vi "NIIE_SET_ToolGraphic.vi"(8 "Error":errorcluster, 9 "Temp Coord":T5, 10 "Temp Icon":picture, 11 "Data":T1={"Class"={"Ants"=refnum, "Layer"=refnum, "Templates"=refnum, "Icon"=refnum, "Glyph"=refnum, "Settings"=refnum, "Tools"=refnum}, "Ref"={"Add Layer"=refnum, "Remove Layer"=refnum, "Line Text"=[], "Body Text Spec"=refnum, "DNL_Font"=refnum, "glyph path str"=refnum, "templates path str"=refnum, "Arrow Up"=refnum, "Arrow Down"=refnum, "IE VI Ref"=refnum, "Glyphs tree"=refnum, "Templates tree"=refnum, "Layer Icon Text"=refnum, "Layer Template"=refnum, "Clipboard"=refnum, "BW icon in"=refnum, "Color icon in"=refnum, "Layer Clust"=refnum, "Body Text"=refnum, "DNL_Framework Templates"=refnum, "Search Templates"=refnum, "TextMarker"=refnum, "Tab Control"=refnum, "Search Glyphs"=refnum, "Line Color"=refnum, "DNL_Glyphs []"=refnum, "Fill Color"=refnum, "Tools"=refnum, "Glyphs tree"=refnum, "Icon"=refnum, "Preview"=refnum, "Ants"=refnum, "Terminals"=refnum, "menu reference"=refnum, "LayerNames"=[], "GlyphLoadAnimation"=refnum, "TemplateLoadAnimation"=refnum, "refreshGlyphs"=refnum, "refreshTemplates"=refnum}, "Support"={"AntsRect"={"left"=0, "top"=0, "right"=0, "bottom"=0}, "Mouse Move Coords"={"Horizontal"=0, "Vertical"=0}, "Mouse Down Coords"={"Horizontal"=0, "Vertical"=0}, "Temp Coord"={"Horizontal"=0, "Vertical"=0}, "Action"=enum."Default", "Edge Color"=4914962, "Fill Color"=16860, "Mouse Down?"=FALSE, "Draft Mode?"=FALSE, "Temp Icon"=bytes[3102], "CTRL Pressed"=FALSE, "Move Selection?"=FALSE, "AntsRect Orig"={"left"=0, "top"=0, "right"=0, "bottom"=0}, "Text"="", "TM Set?"=FALSE, "Mouse inside icon?"=FALSE, "Tool (old value)"=0, "Pencil Move Color"=0, "Swap Colors?"=FALSE, "Shift pressed?"=FALSE}}) -> (0 "Error Out":errorcluster, 1 "All Layers Out":refnum<class "Layer.lvclass">[](array[class]), 3 "Data Out":T1={"Class"={"Ants"=refnum, "Layer"=refnum, "Templates"=refnum, "Icon"=refnum, "Glyph"=refnum, "Settings"=refnum, "Tools"=refnum}, "Ref"={"Add Layer"=refnum, "Remove Layer"=refnum, "Line Text"=[], "Body Text Spec"=refnum, "DNL_Font"=refnum, "glyph path str"=refnum, "templates path str"=refnum, "Arrow Up"=refnum, "Arrow Down"=refnum, "IE VI Ref"=refnum, "Glyphs tree"=refnum, "Templates tree"=refnum, "Layer Icon Text"=refnum, "Layer Template"=refnum, "Clipboard"=refnum, "BW icon in"=refnum, "Color icon in"=refnum, "Layer Clust"=refnum, "Body Text"=refnum, "DNL_Framework Templates"=refnum, "Search Templates"=refnum, "TextMarker"=refnum, "Tab Control"=refnum, "Search Glyphs"=refnum, "Line Color"=refnum, "DNL_Glyphs []"=refnum, "Fill Color"=refnum, "Tools"=refnum, "Glyphs tree"=refnum, "Icon"=refnum, "Preview"=refnum, "Ants"=refnum, "Terminals"=refnum, "menu reference"=refnum, "LayerNames"=[], "GlyphLoadAnimation"=refnum, "TemplateLoadAnimation"=refnum, "refreshGlyphs"=refnum, "refreshTemplates"=refnum}, "Support"={"AntsRect"={"left"=0, "top"=0, "right"=0, "bottom"=0}, "Mouse Move Coords"={"Horizontal"=0, "Vertical"=0}, "Mouse Down Coords"={"Horizontal"=0, "Vertical"=0}, "Temp Coord"={"Horizontal"=0, "Vertical"=0}, "Action"=enum."Default", "Edge Color"=4914962, "Fill Color"=16860, "Mouse Down?"=FALSE, "Draft Mode?"=FALSE, "Temp Icon"=bytes[3102], "CTRL Pressed"=FALSE, "Move Selection?"=FALSE, "AntsRect Orig"={"left"=0, "top"=0, "right"=0, "bottom"=0}, "Text"="", "TM Set?"=FALSE, "Mouse inside icon?"=FALSE, "Tool (old value)"=0, "Pencil Move Color"=0, "Swap Colors?"=FALSE, "Shift pressed?"=FALSE}})   [LabVIEW 2021]
uses:
  <vilib>/Utility/miscctls.llb/LVPoint32TypeDef.ctl
  vi.lib/LabVIEW Icon API/lv_icon/Classes/Layer/Layer.lvclass
  Controls/IE Data.ctl
  Class/Ants/Ants.lvclass
  Class/FakedArray/FakedArray.lvclass
  Class/Icon Library/Glyph.lvclass
  Class/Settings/Settings.lvclass
  Class/Tools/Tools Paint.lvclass
  vi.lib/LabVIEW Icon API/lv_icon/Classes/Icon/Icon.lvclass
  Controls/IE Classes.ctl
  Controls/References Cluster.ctl
  Controls/SupportClass.ctl
  Controls/ENUM_SupportClass_Action.ctl
  vi.lib/LabVIEW Icon API/lv_icon/Controls/IEColor.ctl
  vi.lib/LabVIEW Icon API/lv_icon/Controls/LayerType.ctl
panel:
  in  "FileName":string="Tool"
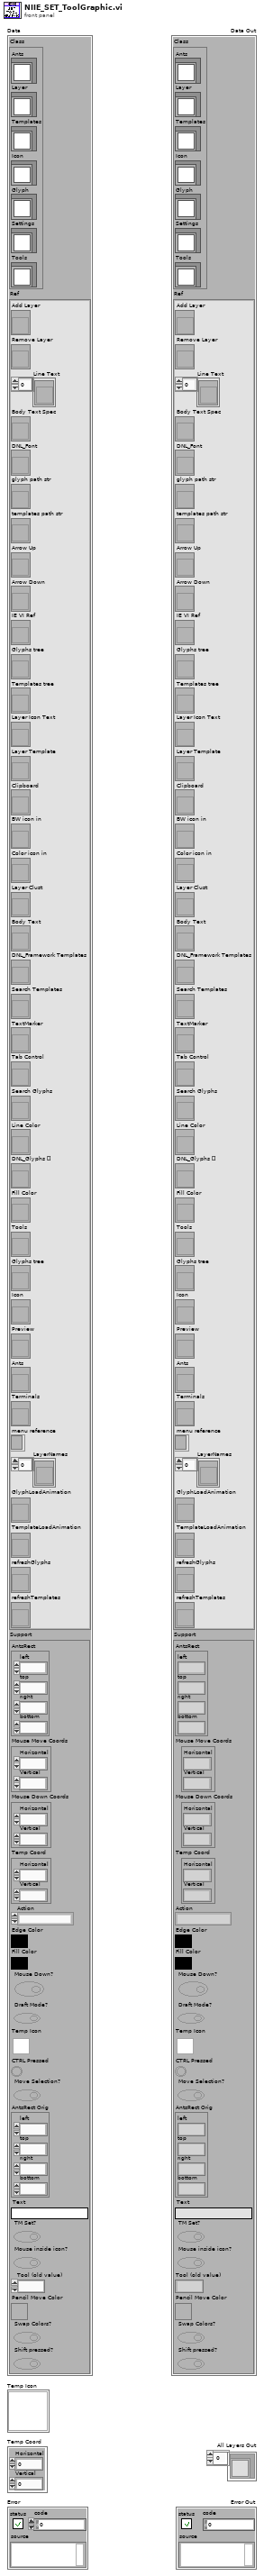
[diagram p1: front panel]
types:
  T1 = typedef "IE Data.ctl" = cluster{"Class":T2, "Ref":T3, "Support":T4}
  T2 = typedef "IE Classes.ctl" = cluster{"Ants":refnum<class "Ants.lvclass">, "Layer":refnum<class "FakedArray.lvclass">, "Templates":refnum<class "FakedArray.lvclass">, "Icon":refnum<class "Icon.lvclass">, "Glyph":refnum<class "Glyph.lvclass">, "Settings":refnum<class "Settings.lvclass">, "Tools":refnum<class "Tools Paint.lvclass">}
  T3 = typedef "References Cluster.ctl" = cluster{"Add Layer":refnum<vi>, "Remove Layer":refnum<vi>, "Line Text":refnum<vi>[], "Body Text Spec":refnum<vi>, "DNL_Font":refnum<vi>, "glyph path str":refnum<vi>, "templates path str":refnum<vi>, "Arrow Up":refnum<vi>, "Arrow Down":refnum<vi>, "IE VI Ref":refnum<vi>, "Glyphs tree":refnum<vi>, "Templates tree":refnum<vi>, "Layer Icon Text":refnum<vi>, "Layer Template":refnum<vi>, "Clipboard":refnum<vi>, "BW icon in":refnum<vi>, "Color icon in":refnum<vi>, "Layer Clust":refnum<vi>, "Body Text":refnum<vi>, "DNL_Framework Templates":refnum<vi>, "Search Templates":refnum<vi>, "TextMarker":refnum<vi>, "Tab Control":refnum<vi>, "Search Glyphs":refnum<vi>, "Line Color":refnum<vi>, "DNL_Glyphs []":refnum<vi>, "Fill Color":refnum<vi>, "Tools":refnum<vi>, "Glyphs tree":refnum<vi>, "Icon":refnum<vi>, "Preview":refnum<vi>, "Ants":refnum<vi>, "Terminals":refnum<vi>, "menu reference":refnum<k9>, "LayerNames":refnum<vi>[], "GlyphLoadAnimation":refnum<vi>, "TemplateLoadAnimation":refnum<vi>, "refreshGlyphs":refnum<vi>, "refreshTemplates":refnum<vi>}
  T4 = typedef "SupportClass.ctl" = cluster{"AntsRect":cluster{"left":i16, "top":i16, "right":i16, "bottom":i16}, "Mouse Move Coords":T5, "Mouse Down Coords":T5, "Temp Coord":T5, "Action":T6, "Edge Color":T7, "Fill Color":T7, "Mouse Down?":bool, "Draft Mode?":bool, "Temp Icon":picture, "CTRL Pressed":bool, "Move Selection?":bool, "AntsRect Orig":cluster{"left":i16, "top":i16, "right":i16, "bottom":i16}, "Text":string, "TM Set?":bool, "Mouse inside icon?":bool, "Tool (old value)":u32, "Pencil Move Color":u32, "Swap Colors?":bool, "Shift pressed?":bool}
  T5 = typedef "LVPoint32TypeDef.ctl" = cluster{"Horizontal":i32, "Vertical":i32}
  T6 = typedef "ENUM_SupportClass_Action.ctl" = enum16{"Default", "Move Selection", "Glyph Library", "Tool"}
  T7 = typedef "IEColor.ctl" = u32
  T8 = cluster{"left":i16, "top":i16, "right":i16, "bottom":i16}
  T9 = typedef "Cluster_INI Data.ctl" = cluster{"Show Layer Tab?":bool, "Show Terminals?":bool, "Text":cluster{"Font":T10, "Alignment":T11, "Size":T12}, "3rd party Templates":cluster{"Store 3rd party Templates?":bool, "Folder Name":string}, "Merge user layers on commit":bool, "Body Text":T13, "Fill Color":T7, "Edge Color":T7, "Tab":u16, "Tool":T14, "Disable Layers?":bool}
  T10 = typedef "Font.ctl" = string
  T11 = typedef "Alignment.ctl" = u16
  T12 = typedef "Num_Font Size.ctl" = u8
  T13 = typedef "Cluster_BodyText.ctl" = cluster{"Line 1 text":string, "Line 2 text":string, "Line 3 text":string, "Line 4 text":string, "Line 1 color":u32, "Line 2 color":u32, "Line 3 color":u32, "Line 4 color":u32, "Body Text Spec":cluster{"Font":T10, "Alignment":T11, "Size":u8}, "Center text vertically":bool, "Capitalize Text":bool}
  T14 = typedef "Cluster_Button Draw Tools.ctl" = enum32{"Pencil", "Line", "Dropper", "Fill", "Rectangle", "Filled Rectangle", "Ellipse", "Filled Ellipse", "Eraser", "Text", "Select", "Move"}
  T15 = typedef "LayerType.ctl" = enum16{"Graphic", "Text", "Tool", "Graphic Drop"}
  T16 = typedef "Cluster_Layer Data.ctl" = cluster{"LayerIcon":picture, "LayerName":string, "Opacity":u8, "Visibility?":bool}
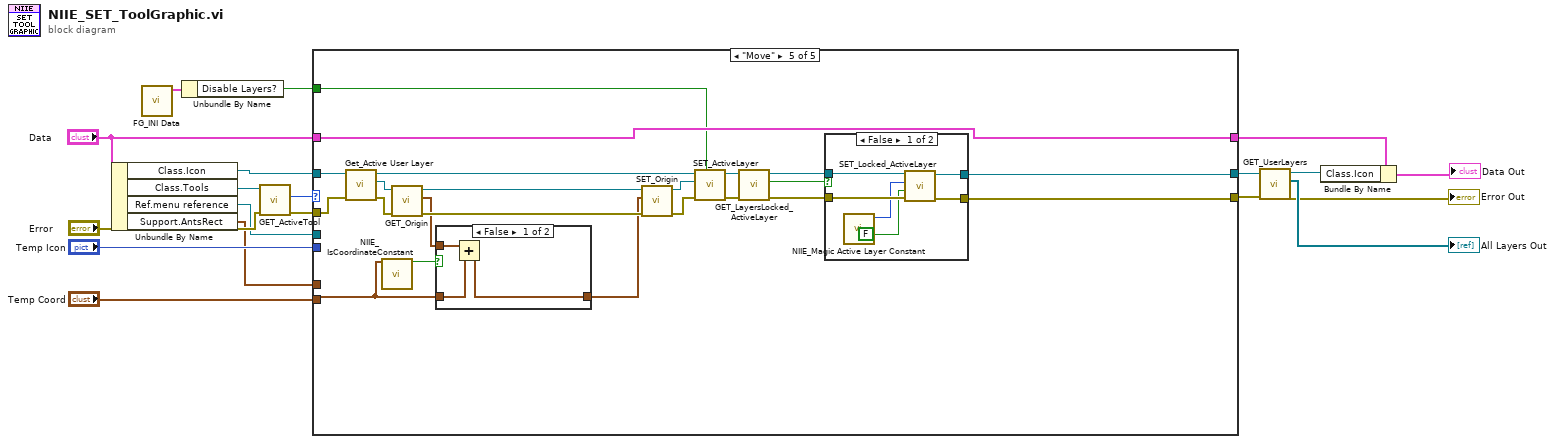
[diagram p0: block diagram]
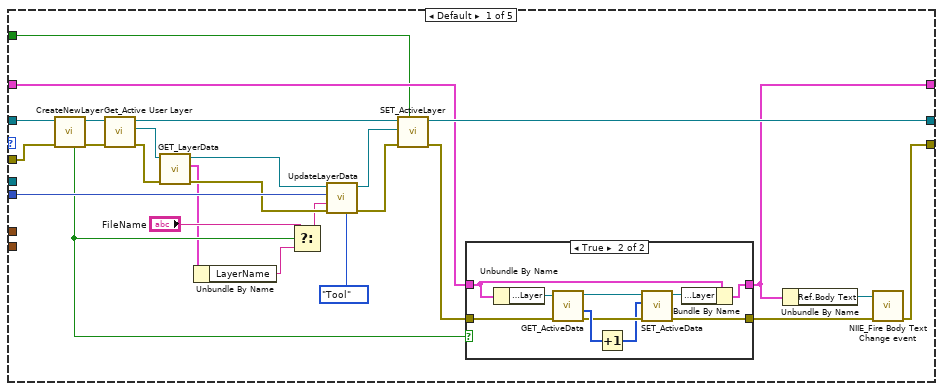
[diagram p2: hidden frame]
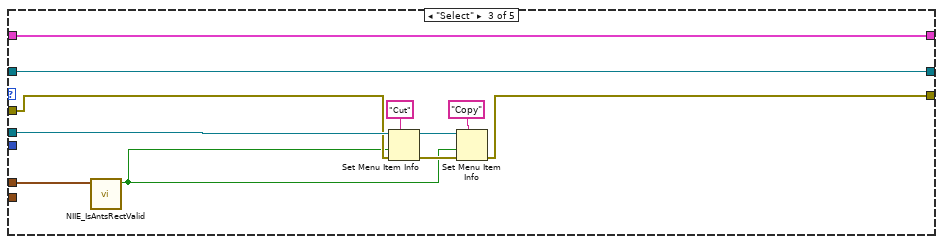
[diagram p5: hidden frame]
diagram:
  n1 = Unbundle By Name("Data") -> ("Class.Icon"=w11:refnum<class "Icon.lvclass">, "Class.Tools"=w12:refnum<class "Tools Paint.lvclass">, "Ref.menu reference"=w4:refnum<k9>, "Support.AntsRect"=w3:T8)
  n2 = call "FG_INI Data.vi"() -> ("INI Data Out"=w2:T9)  [unwired: 9 in, 2 out]
  n3 = Unbundle By Name(w2) -> ("Disable Layers?"=w1:bool)
  n4 = call-dynamic "GET_ActiveTool.vi"("error in (no error)"="Error", "Tools Paint.lvclass in"=w12) -> ("error out"=w14:errorcluster, "Radio Buttons"=w13:T14)  [unwired: 8 out]
  n5 = case shown="\"Move\"" w13 {
    tunnel: w11 -> [w45 w60 w71 w74 w95]
    tunnel: "Temp Icon" -> [w39 _ _ _ _]
    tunnel: [w38 w60 w71 w74 w79] -> w18
    tunnel: [w21 w59 w63 w73 w78] -> w19
    tunnel: "Temp Coord" -> [_ _ _ _ w86]
    tunnel: w14 -> [w36 w59 w64 w73 w77]
    tunnel: "Data" -> [w25 w58 w70 w72 w76]
    tunnel: [w24 w58 w70 w72 w76] -> w8
    tunnel: w4 -> [_ _ w65 _ _]
    tunnel: w3 -> [_ _ w62 _ _]
    tunnel: w1 -> [w20 _ _ _ w75]
    frame Default {
      n6 = call "CreateNewLayer.vi"("error in"=w36, "Icon.lvclass"=w45) -> ("error out"=w43:errorcluster, "Icon.lvclass out"=w44:refnum<class "Icon.lvclass">, "Layer added?"=w34:bool)  [unwired: 3 in, 4 out]
      n7 = call-dynamic "Get_Active User Layer.vi"("error in (no error)"=w43, "Icon in"=w44) -> ("error out"=w32:errorcluster, "Layer.lvclass"=w30:refnum<class "Layer.lvclass">, "Icon out"=w42:refnum<class "Icon.lvclass">)  [unwired: 7 out]
      n8 = call-dynamic "GET_LayerData.vi"("error in (no error)"=w32, "Layer.lvclass in"=w30) -> ("error out"=w31:errorcluster, "Data"=w28:T16, "Layer.lvclass out"=w29:refnum<class "Layer.lvclass">)  [unwired: 7 out]
      n9 = Unbundle By Name(w28) -> ("LayerName"=w27:string)
      n10 = Select(t="FileName", s=w34, f=w27) -> (s? t:f=w26:string)
      n11 = call "UpdateLayerData.vi"("Type"=LayerType."Tool", "error in"=w31, "LayerName"=w26, "new picture"=w39, "Active Layer"=w29) -> ("error out"=w40:errorcluster, "Layer.lvclass out"=w41:refnum<class "Layer.lvclass">)  [unwired: 3 in, 2 out]
      n12 = call-dynamic "SET_ActiveLayer.vi"("Combine User Layers?"=w20, "Error"=w40, "Layer.lvclass"=w41, "Icon.lvclass"=w42) -> ("Error Out"=w35:errorcluster, "Icon.lvclass Out"=w38:refnum<class "Icon.lvclass">)  [unwired: 6 out]
      n13 = case shown="True" w34 {
        tunnel: w35 -> [w47 w48]
        tunnel: [w47 w50] -> w22
        tunnel: w25 -> [w46 w52]
        tunnel: [w46 w49] -> w24
        frame False {
        }
        frame True {
          n14 = Unbundle By Name(w52) -> ("Class.Layer"=w53:refnum<class "FakedArray.lvclass">)
          n15 = call-dynamic "GET_ActiveData.vi"("Error"=w48, "FakedArray"=w53) -> ("Error Out"=w55:errorcluster, "Active Data [] Out"=w56:i32[], "FakedArray Out"=w57:refnum<class "FakedArray.lvclass">)  [unwired: 7 out]
          n16 = Increment(x=w56) -> (x+1=w54:i32[])
          n17 = call-dynamic "SET_ActiveData.vi"("error in (no error)"=w55, "Active Data"=w54, "FakedArray.lvclass in"=w57) -> ("error out"=w50:errorcluster, "FakedArray.lvclass out"=w51:refnum<class "FakedArray.lvclass">)  [unwired: 7 out]
          n18 = Bundle By Name(cluster=w52, "Class.Layer"=w51) -> (w49:T1)
        }
      }
      n19 = Unbundle By Name(w24) -> ("Ref.Body Text"=w23:refnum<vi>)
      n20 = call "NIIE_Fire Body Text Change event.vi"("error in"=w22, "Ref.Body Text"=w23) -> ("error out"=w21:errorcluster)  [unwired: 2 in, 7 out]
    }
    frame "Fill" {
    }
    frame "Select" {
      n21 = call "NIIE_IsAntsRectValid.vi"("Image Range"=w62) -> ("Valid? Out"=w61:bool)  [unwired: 10 out]
      n22 = Set Menu Item Info(7:"Cut" ("item tag"), 8:w64, 9:w61, 11:w65) -> (0:w69:errorcluster, 3:w67:refnum<k9>)  [unwired: 3 out]
      n23 = Set Menu Item Info(7:"Copy" ("item tag"), 8:w69, 9:w61, 11:w67) -> (0:w63:errorcluster)  [unwired: 4 out]
    }
    frame "Dropper", "Eraser" {
    }
    frame "Move" {
      n24 = call-dynamic "Get_Active User Layer.vi"("error in (no error)"=w77, "Icon in"=w95) -> ("error out"=w90:errorcluster, "Layer.lvclass"=w92:refnum<class "Layer.lvclass">, "Icon out"=w96:refnum<class "Icon.lvclass">)  [unwired: 7 out]
      n25 = call "NIIE_IsCoordinateConstant.vi"("Coordinate"=w86) -> ("Constant?"=w85:bool)  [unwired: 10 out]
      n26 = call-dynamic "GET_Origin.vi"("error in (no error)"=w90, "Layer.lvclass in"=w92) -> ("error out"=w89:errorcluster, "Point32"=w88:T5, "Layer.lvclass out"=w91:refnum<class "Layer.lvclass">)  [unwired: 7 out]
      n27 = case shown="False" w85 {
        tunnel: w88 -> [w107 w108]
        tunnel: [w105 w108] -> w87
        tunnel: w86 -> [w106 _]
        frame False {
          n28 = Add(x=w107, y=w106) -> (x+y=w105:T5)
        }
        frame True {
        }
      }
      n29 = call-dynamic "SET_Origin.vi"("error in (no error)"=w89, "Point32"=w87, "Layer.lvclass in"=w91) -> ("error out"=w93:errorcluster, "Layer.lvclass out"=w94:refnum<class "Layer.lvclass">)  [unwired: 7 out]
      n30 = call-dynamic "SET_ActiveLayer.vi"("Combine User Layers?"=w75, "Error"=w93, "Layer.lvclass"=w94, "Icon.lvclass"=w96) -> ("Error Out"=w84:errorcluster, "Icon.lvclass Out"=w83:refnum<class "Icon.lvclass">)  [unwired: 6 out]
      n31 = call-dynamic "GET_LayersLocked_ActiveLayer.vi"("error in (no error)"=w84, "Icon.lvclass in"=w83) -> ("error out"=w80:errorcluster, "Layers Locked?"=w82:bool, "Icon.lvclass out"=w81:refnum<class "Icon.lvclass">)  [unwired: 7 out]
      n32 = case shown="False" w82 {
        tunnel: w81 -> [w102 w104]
        tunnel: w80 -> [w101 w103]
        tunnel: [w99 w104] -> w79
        tunnel: [w98 w103] -> w78
        frame False {
          n33 = call "NIIE_Magic Active Layer Constant.vi"() -> ("Magic Constant"=w97:i32)  [unwired: 11 in]
          n34 = call-dynamic "SET_Locked_ActiveLayer.vi"("error in (no error)"=w101, "Layers Locked?"=FALSE, "Active Layer"=w97, "Icon.lvclass in"=w102) -> ("error out"=w98:errorcluster, "Icon.lvclass out"=w99:refnum<class "Icon.lvclass">)  [unwired: 6 out]
        }
        frame True {
        }
      }
    }
  }
  n35 = call-dynamic "GET_UserLayers.vi"("error in (no error)"=w19, "Icon.lvclass in"=w18) -> ("error out"=→"Error Out":errorcluster, "All Layers"=→"All Layers Out":refnum<class "Layer.lvclass">[], "Icon.lvclass out"=w7:refnum<class "Icon.lvclass">)  [unwired: 7 out]
  n36 = Bundle By Name(cluster=w8, "Class.Icon"=w7) -> (→"Data Out":T1)
